vi "GOOP_LVClass_Global_Interface.vi"() -> (3 "InterfaceTable":T1)   [LabVIEW 2012]
doc: "NI Confidential \n\n/**\n@brief This VI tells the framework which VIs to call when an event happens related to one of your items.\n\n@author Joel Dixon\n\n@par Sample_Item_Interface.vi\n For each of the entries in the InterfaceTable, pass in a string representing a relative path to a VI which implements that method. Methods include Init, Exit, OnCommand, OnDropFiles, and OnSelect. \n\n@param \"InterfaceTable\" [out] \nThis is an array of strings passed back to the framework so it knows which VIs should be called under what circumstances.\n*/"
uses:
  <resource>/Framework/Providers/API/Global_Interface.ctl
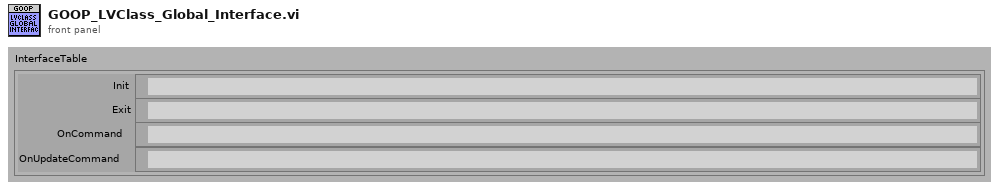
[diagram p1: front panel]
types:
  T1 = typedef "Global_Interface.ctl" = cluster{"Init":path, "Exit":path, "OnCommand":path, "OnUpdateCommand":path}
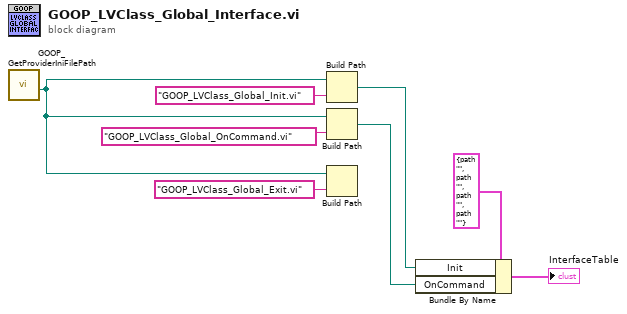
[diagram p0: block diagram]
diagram:
  n1 = call <resource>:"GOOP_GetProviderIniFilePath.vi"() -> ("ProviderMainFolder"=w2:path)  [unwired: 10 in, 1 out]
  n2 = Build Path(base path=w2, name or relative path="GOOP_LVClass_Global_Init.vi") -> (appended path=w4:path)
  n3 = Build Path(base path=w2, name or relative path="GOOP_LVClass_Global_OnCommand.vi") -> (appended path=w1:path)
  n4 = Build Path(base path=w2, name or relative path="GOOP_LVClass_Global_Exit.vi") -> ()  [unwired: 1 out]
  n5 = Bundle By Name(cluster=T1 {"Init"=path "", "Exit"=path "", "OnCommand"=path "", "OnUpdateCommand"=path ""} ("InterfaceTable"), "Init"=w4, "OnCommand"=w1) -> (→"InterfaceTable":T1)
